vi "CONV_ANGLES.vi"(8 "error in (no error)":errorcluster, 9 "IN (DEG)":dbl, 10 "IN (RAD)":dbl, 11 "reference in":refnum<class "Manipulator.lvclass">) -> (0 "error out":errorcluster, 1 "OUT (RAD)":dbl, 2 "OUT (DEG)":dbl, 3 "reference out":refnum<class "Manipulator.lvclass">)   [LabVIEW 2014, in "Manipulator.lvclass"]
uses:
  Manipulator.lvclass
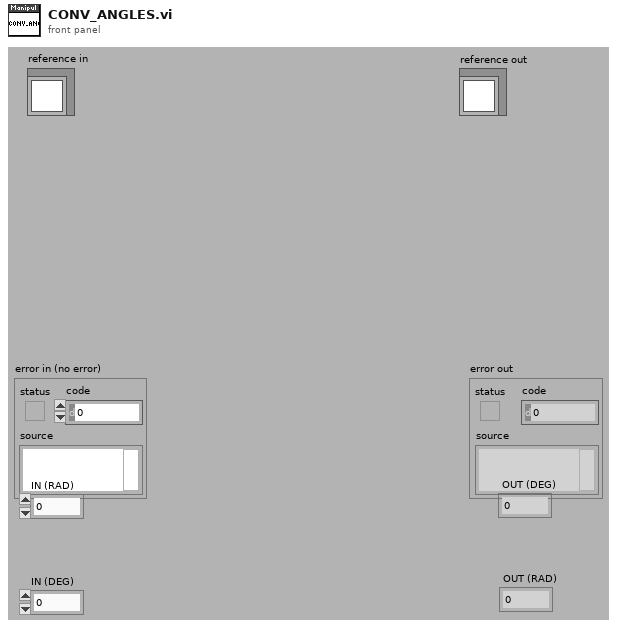
[diagram p1: front panel]
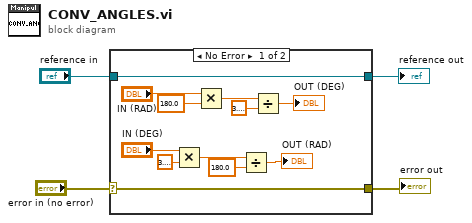
[diagram p0: block diagram]
diagram:
  n1 = case shown="No Error" "error in (no error)" {
    selector: "error in (no error)" -> [w5 w18]
    tunnel: [w5 w18] -> w3
    tunnel: [w6 w17] -> w1
    tunnel: "reference in" -> [w6 w17]
    frame No Error {
      n2 = Multiply(x="IN (DEG)", y=3.141592653589793) -> (x*y=w9:dbl)
      n3 = Multiply(x="IN (RAD)", y=180.0) -> (x*y=w14:dbl)
      n4 = Divide(x=w9, y=180.0) -> (x/y=→"OUT (RAD)":dbl)
      n5 = Divide(x=w14, y=3.141592653589793) -> (x/y=→"OUT (DEG)":dbl)
    }
    frame Error {
    }
  }
  "error out" <- w3
  "reference out" <- w1
